vi "ALTS-2015 Write Robot Task v0.1.vi"(8 "error in (no error)":errorcluster, 11 "Task Details":T4) -> (0 "error out":errorcluster, 3 "Next State to Execute":T3=enum."Wait for Robot Availability", 5 "Last Robot Task":T2, 7 "Last Robot Task Out Station #":T1)   [LabVIEW 2013]
uses:
  Controls/ALTS-2015 Auto Program States.ctl
  Controls/ALTS-2015 LV2GBL Station Info Options.ctl
  Controls/ALTS-2015 Status Ring Indicator.ctl
  Controls/ALTS-2015 Station Details.ctl
  Controls/ALTS-2015 Write Robot Task OPC Options.ctl
  Controls/ALTS-2015 Robot FIFO Queue Options.ctl
  Controls/ALTS-2015 Robot Tasks.ctl
  Controls/ALTS-2015 Robot Actions.ctl
  Controls/ALTS-2015 Station Cluster.ctl
  Controls/ALTS-2015 Serial Details.ctl
  Controls/ALTS-2015 Serial DB Details.ctl
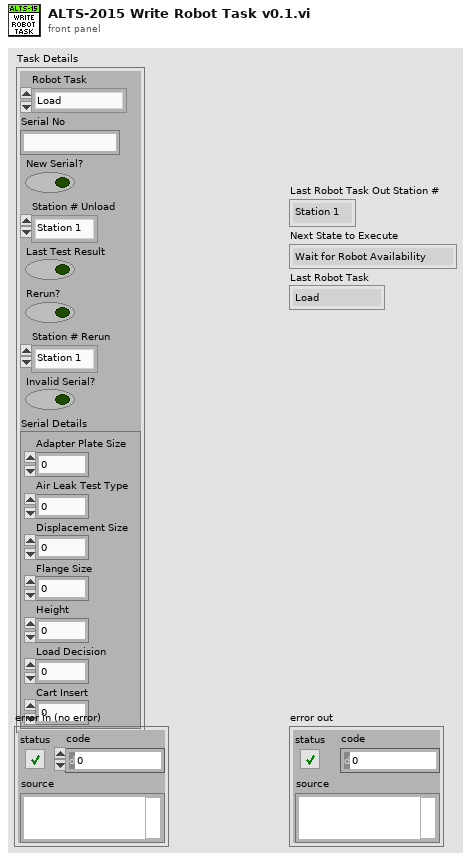
[diagram p1: front panel]
types:
  T1 = typedef "ALTS-2015 Station Cluster.ctl" = enum16{"Station 1", "Station 2", "Station 3", "Station 4"}
  T2 = typedef "ALTS-2015 Robot Tasks.ctl" = enum16{"Load", "Unload", "Rerun", "Invalid Serial"}
  T3 = typedef "ALTS-2015 Auto Program States.ctl" = enum16{"<------ Robot Handler States ------>", "Wait for Robot Availability", "Check Last Task by Robot", "Wait & Read Task from Queue", "Write New Task Details to Robot", "Write Task Available for Robot", "Check Robot for Unavailbilty", "Write Task Unavailable for Robot", "<------------ Other ------------>", "Error", "Exit"}
  T4 = typedef "ALTS-2015 Serial Details.ctl" = cluster{"Robot Task":T2, "Serial No":string, "New Serial?":bool, "Station # Unload":T1, "Last Test Result":bool, "Rerun?":bool, "Station # Rerun":T1, "Invalid Serial?":bool, "Serial Details":T5}
  T5 = typedef "ALTS-2015 Serial DB Details.ctl" = cluster{"Adapter Plate Size":i32, "Air Leak Test Type ":i32, "Displacement Size":i32, "Flange Size":i32, "Height":i32, "Load Decision":i32, "Cart Insert":i32}
  T6 = typedef "ALTS-2015 Robot Actions.ctl" = enum16{"Loading...", "Unloading...", "Reruning...", "No Action"}
  T7 = typedef "ALTS-2015 Station Details.ctl" = cluster{"Station Number":string, "Work Order Number":string, "Sensor Name":string, "Pressure (PSI)":string, "Flow (SCCM)":string, "Test Time ":string, "Test Result":string, "Serial Number":string, "Station Status":T8, "SW assigned UUT":bool, "Rerun Count":i32, "Test Type":i32, "Load Decision":i32, "Robot Action":T6}
  T8 = typedef "ALTS-2015 Status Ring Indicator.ctl" = u16
  T9 = typedef "ALTS-2015 Write Robot Task OPC Options.ctl" = enum16{"Write New Serial Task", "Write Rerun Task", "Write Unload Task", "Write Invalid Serial Task"}
  T10 = typedef "ALTS-2015 Robot FIFO Queue Options.ctl" = enum16{"Init", "Enqueue", "Dequeue", "Get Queue Elements", "Flush", "Destroy"}
  T11 = typedef "ALTS-2015 LV2GBL Station Info Options.ctl" = enum16{"Init", "Read", "Read All", "Write Sensor ID", "Write  Work Order", "Write Serial Number", "Write Test Data", "Write Station Status", "Write Station Occupancy", "Write Station Test Type", "Write Rerun", "Write Load Decision", "Write Robot Action", "Clear All", "Clear Test Result"}
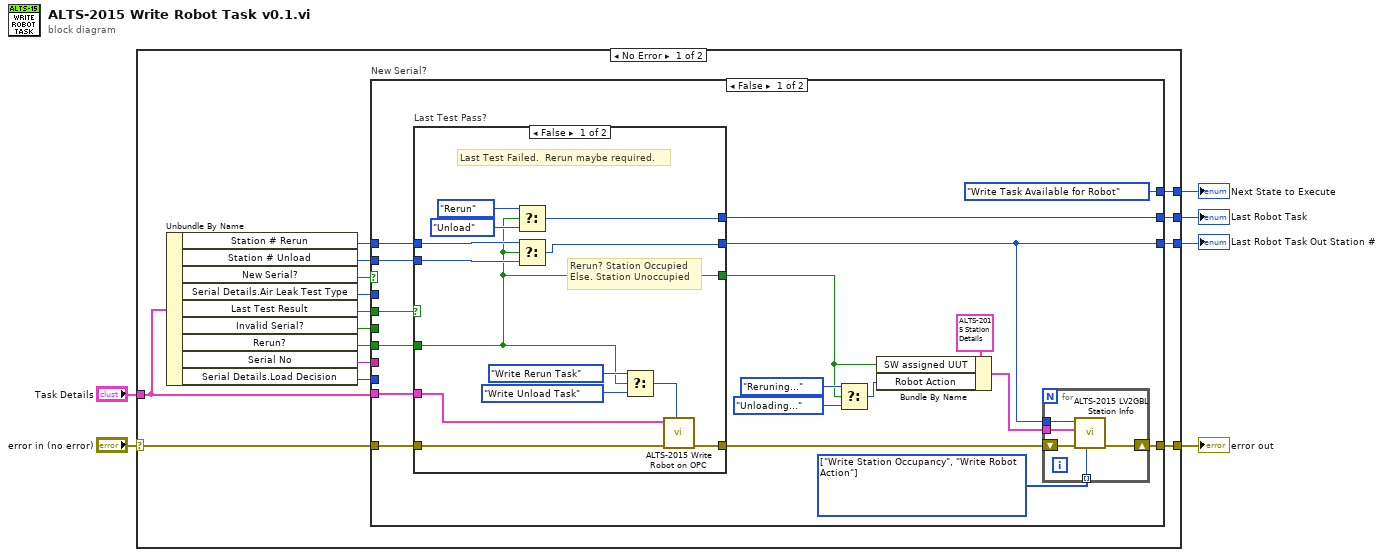
[diagram p0: block diagram]
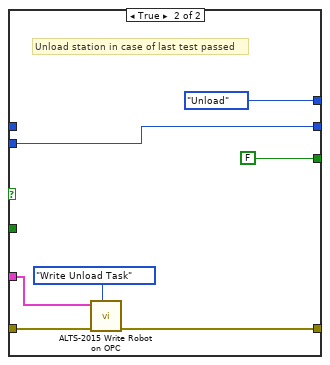
[diagram p2: hidden frame]
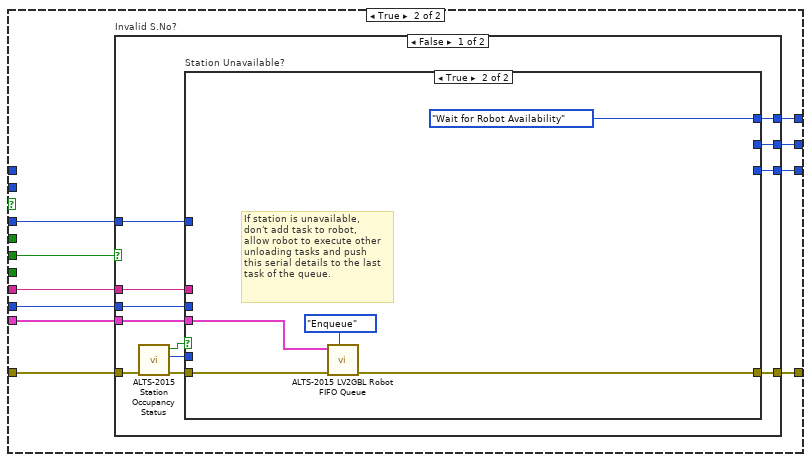
[diagram p3: hidden frame]
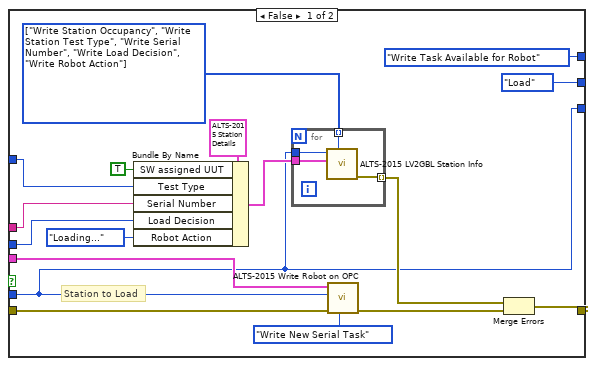
[diagram p4: hidden frame]
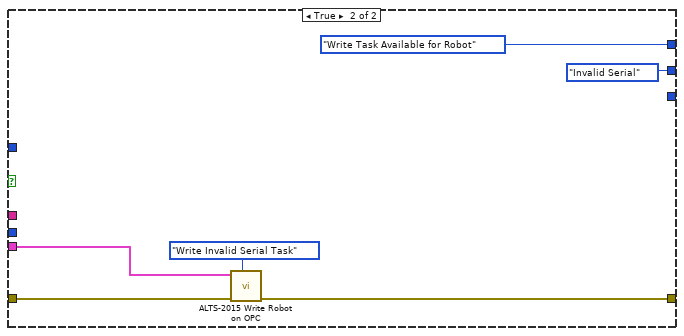
[diagram p5: hidden frame]
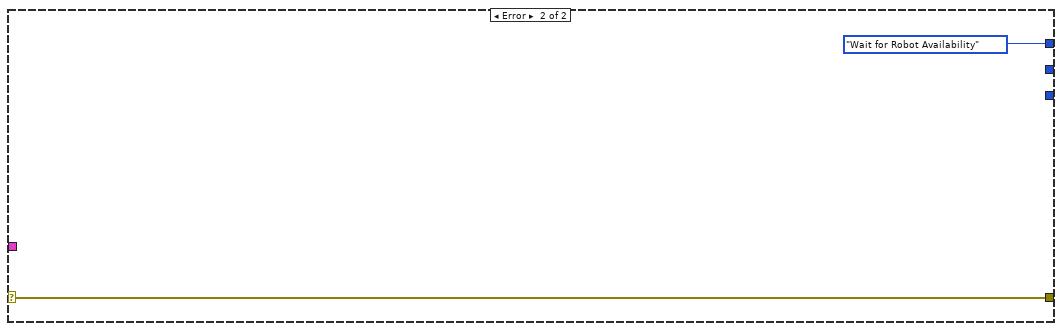
[diagram p6: hidden frame]
diagram:
  n1 = case shown="No Error" "error in (no error)" {
    selector: "error in (no error)" -> [w11 w120]
    tunnel: [w20 ALTS-2015_Auto_Program_States."Wait for Robot Availability"] -> w6
    tunnel: [w18 w120] -> w5
    tunnel: "Task Details" -> [w17 _]
    tunnel: [w8 _] -> w2
    tunnel: [w7 _] -> w1
    frame No Error {
      n2 = Unbundle By Name(w17) -> ("Station # Rerun"=w12:T1, "Station # Unload"=w13:T1, "New Serial?"=w19:bool, "Serial Details.Air Leak Test Type"=w16:i32, "Last Test Result"=w15:bool, "Invalid Serial?"=w21:bool, "Rerun?"=w14:bool, "Serial No"=w10:string, "Serial Details.Load Decision"=w9:i32)
      n3 = case "New Serial?" shown="False" w19 {
        tunnel: [ALTS-2015_Auto_Program_States."Write Task Available for Robot" w71] -> w20
        tunnel: [w27 w74] -> w18
        tunnel: w11 -> [w36 w73]
        tunnel: w17 -> [w34 w72]
        tunnel: w21 -> [_ w70]
        tunnel: w16 -> [_ w69]
        tunnel: w15 -> [w35 _]
        tunnel: w14 -> [w33 _]
        tunnel: w13 -> [w31 _]
        tunnel: w12 -> [w32 _]
        tunnel: w10 -> [_ w68]
        tunnel: w9 -> [_ w67]
        tunnel: [w30 w66] -> w8
        tunnel: [w28 w65] -> w7
        frame False {
          w26 = T11[] [enum."Write Station Occupancy", enum."Write Robot Action"] items=["Init", "Read", "Read All", "Write Sensor ID", "Write  Work Order", "Write Serial Number", "Write Test Data", "Write Station Status", "Write Station Occupancy", "Write Station Test Type", "Write Rerun", "Write Load Decision", "Write Robot Action", "Clear All", "Clear Test Result"]
          n4 = case "Last Test Pass?" shown="False" w35 {
            tunnel: [w45 FALSE ("Rerun?")] -> w22
            tunnel: w34 -> [w57 w61]
            tunnel: w36 -> [w56 w63]
            tunnel: [w55 w62] -> w29
            tunnel: w33 -> [w45 _]
            tunnel: [w46 w59] -> w28
            tunnel: w32 -> [w48 _]
            tunnel: w31 -> [w47 w59]
            tunnel: [w52 ALTS-2015_Robot_Tasks."Unload" ("Last Robot Task")] -> w30
            frame False {
              # "Rerun? Station Occupied\nElse. Station Unoccupied"
              # "Last Test Failed.  Rerun maybe required."
              n5 = Select(t=ALTS-2015_Robot_Tasks."Rerun" ("Last Robot Task"), s=w45, f=ALTS-2015_Robot_Tasks."Unload" ("Last Robot Task")) -> (s? t:f=w52:T2)
              n6 = Select(t=w48, s=w45, f=w47) -> (s? t:f=w46:T1)
              n7 = Select(t=ALTS-2015_Write_Robot_Task_OPC_Options."Write Rerun Task" ("Option"), s=w45, f=ALTS-2015_Write_Robot_Task_OPC_Options."Write Unload Task" ("Option")) -> (s? t:f=w49:T9)
              n8 = call "ALTS-2015 Write Robot on OPC.vi"("Option"=w49, "error in (no error)"=w56, "Serial Details in"=w57) -> ("error out"=w55:errorcluster)  [unwired: 8 in]
            }
            frame True {
              # "Unload station in case of last test passed"
              n9 = call "ALTS-2015 Write Robot on OPC.vi"("Option"=ALTS-2015_Write_Robot_Task_OPC_Options."Write Unload Task", "error in (no error)"=w63, "Serial Details in"=w61) -> ("error out"=w62:errorcluster)  [unwired: 8 in]
            }
          }
          n10 = Select(t=ALTS-2015_Robot_Actions."Reruning...", s=w22, f=ALTS-2015_Robot_Actions."Unloading..." ("Robot Action")) -> (s? t:f=w24:T6)
          n11 = Bundle By Name(cluster=T7 {"Station Number"="", "Work Order Number"="", "Sensor Name"="", "Pressure (PSI)"="", "Flow (SCCM)"="", "Test Time "="", "Test Result"="", "Serial Number"="", "Station Status"=0, "SW assigned UUT"=FALSE, "Rerun Count"=0, "Test Type"=0, "Load Decision"=0, "Robot Action"=enum."Loading..."} ("Station"), "SW assigned UUT"=w22, "Robot Action"=w24) -> (w37:T7)
          n12 = for {
            tunnel: w37 -> [w44]
            tunnel: w28 -> [w42]
            tunnel: w26 -> [w40] mode=indexing
            shift-right: [w41] -> w27
            shift-left: w29 -> [w43]
            n13 = call "ALTS-2015 LV2GBL Station Info.vi"("Options"=w40, "error in"=w43, "Station"=w44, "Station Cluster"=w42) -> ("error out"=w41:errorcluster)  [unwired: 5 in, 2 out]
          }
        }
        frame True {
          n14 = case "Invalid S.No?" shown="False" w70 {
            tunnel: [w84 w116] -> w74
            tunnel: w73 -> [w82 w117]
            tunnel: w72 -> [w81 w115]
            tunnel: [w80 ALTS-2015_Auto_Program_States."Write Task Available for Robot"] -> w71
            tunnel: w69 -> [w79 _]
            tunnel: w68 -> [w78 _]
            tunnel: w67 -> [w77 _]
            tunnel: [w76 ALTS-2015_Robot_Tasks."Invalid Serial" ("Last Robot Task")] -> w66
            tunnel: [w75 _] -> w65
            frame False {
              n15 = call "ALTS-2015 Station Occupancy Status.vi"("error in"=w82) -> ("error out"=w83:errorcluster, "Available Station"=w85:T1, "Station Unavailable"=w86:bool)  [unwired: 8 in]
              n16 = case "Station Unavailable?" shown="True" w86 {
                tunnel: w85 -> [w88 _]
                tunnel: [w92 w110] -> w84
                tunnel: w83 -> [w103 w111]
                tunnel: w81 -> [w98 w109]
                tunnel: [ALTS-2015_Auto_Program_States."Write Task Available for Robot" ALTS-2015_Auto_Program_States."Wait for Robot Availability"] -> w80
                tunnel: w79 -> [w96 _]
                tunnel: w78 -> [w95 _]
                tunnel: w77 -> [w93 _]
                tunnel: [ALTS-2015_Robot_Tasks."Load" ("Last Robot Task") _] -> w76
                tunnel: [w88 _] -> w75
                frame False {
                  w90 = T11[] [enum."Write Station Occupancy", enum."Write Station Test Type", enum."Write Serial Number", enum."Write Load Decision", enum."Write Robot Action"] items=["Init", "Read", "Read All", "Write Sensor ID", "Write  Work Order", "Write Serial Number", "Write Test Data", "Write Station Status", "Write Station Occupancy", "Write Station Test Type", "Write Rerun", "Write Load Decision", "Write Robot Action", "Clear All", "Clear Test Result"]
                  # "Station to Load"
                  n17 = Bundle By Name(cluster=T7 {"Station Number"="", "Work Order Number"="", "Sensor Name"="", "Pressure (PSI)"="", "Flow (SCCM)"="", "Test Time "="", "Test Result"="", "Serial Number"="", "Station Status"=0, "SW assigned UUT"=FALSE, "Rerun Count"=0, "Test Type"=0, "Load Decision"=0, "Robot Action"=enum."Loading..."} ("Station"), "SW assigned UUT"=TRUE ("Rerun?"), "Test Type"=w96, "Serial Number"=w95, "Load Decision"=w93, "Robot Action"=ALTS-2015_Robot_Actions."Loading...") -> (w94:T7)
                  n18 = for {
                    tunnel: w94 -> [w107]
                    tunnel: w88 -> [w106]
                    tunnel: [w105] -> w91 mode=indexing
                    tunnel: w90 -> [w104] mode=indexing
                    n19 = call "ALTS-2015 LV2GBL Station Info.vi"("Options"=w104, "Station"=w107, "Station Cluster"=w106) -> ("error out"=w105:errorcluster)  [unwired: 6 in, 2 out]
                  }
                  n20 = call "ALTS-2015 Write Robot on OPC.vi"("Option"=ALTS-2015_Write_Robot_Task_OPC_Options."Write New Serial Task", "error in (no error)"=w103, "Station # Load"=w88, "Serial Details in"=w98) -> ("error out"=w99:errorcluster)  [unwired: 7 in]
                  n21 = Merge Errors(w91, w99) -> (w92:errorcluster)
                }
                frame True {
                  # "If station is unavailable,\ndon't add task to robot,\nallow robot to execute other\nunloading tasks and push\nthis serial details to the last\ntask of the queue."
                  n22 = call "ALTS-2015 LV2GBL Robot FIFO Queue.vi"("Options"=ALTS-2015_Robot_FIFO_Queue_Options."Enqueue" ("Enum"), "error in (no error)"=w111, "Task Details In"=w109) -> ("error out"=w110:errorcluster)  [unwired: 4 in, 4 out]
                }
              }
            }
            frame True {
              n23 = call "ALTS-2015 Write Robot on OPC.vi"("Option"=ALTS-2015_Write_Robot_Task_OPC_Options."Write Invalid Serial Task", "error in (no error)"=w117, "Serial Details in"=w115) -> ("error out"=w116:errorcluster)  [unwired: 8 in]
            }
          }
        }
      }
    }
    frame Error {
    }
  }
  "Next State to Execute" <- w6
  "error out" <- w5
  "Last Robot Task" <- w2
  "Last Robot Task Out Station #" <- w1
